vi "LSRS CompleteDrive.vi"() -> ()   [LabVIEW 2017]
uses:
  <vilib>/Rock Robotics/Network Tables/NT Write Numeric Array.vi
panel:
  in  "Error In":errorcluster
  out "Error Out":errorcluster
  out "Right Front Motor Output":dbl
  out "Right Back Motor Output":dbl
  out "Left Front Motor Output":dbl
  out "Left Back Motor Output":dbl
  in  "X":dbl
  in  "Y":dbl
  in  "Z":dbl
  in  "Robot Width":dbl=28.5
  in  "Robot Length":dbl=33.5
  in  "Robot Centric?":bool=TRUE
  in  "Rot. Point X":dbl
  in  "Rot. Point Y":dbl
  in  "Autonomous?":bool
  in  "Yaw":dbl
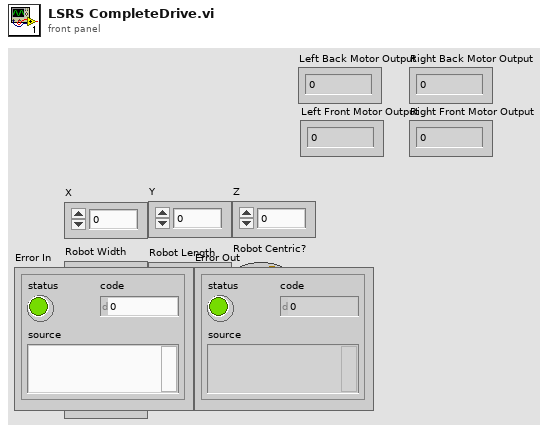
[diagram p1: front panel]
types:
  T1 = typedef "WPI_MotorControlDeviceRef.ctl" = cluster{"DeviceStatus":errorcluster, "Type":T2, "PWM":cluster{"PWM Channel":T3, "DeadBand":T4}, "CAN":cluster{"Device Number":u8, "SetOutput VI Ref":variant, "GetOutput VI Ref":variant, "Enable VI Ref":variant, "Disable VI Ref":variant, "Data":variant}, "Invert":bool, "DIO PWM":cluster{"PWM \"Enable\" Channel":T3, "DIOChannel":T5, "PWM Rate":dbl}}
  T2 = typedef "WPI_MotorControlType.ctl" = enum16{"PWM", "CAN", "DIO PWM"}
  T3 = typedef "FPGA_DIOPWMChannel.ctl" = enum8{"PWM 0", "PWM 1", "PWM 2", "PWM 3", "PWM 4", "PWM 5", "PWM 6", "PWM 7", "PWM 8", "PWM 9", "PWM MXP 0", "PWM MXP 1", "PWM MXP 2", "PWM MXP 3", "PWM MXP 4", "PWM MXP 5", "PWM MXP 6", "PWM MXP 7", "PWM MXP 8", "PWM MXP 9", "Invalid"}
  T4 = typedef "WPI_PWMDeadband.ctl" = cluster{"Name":string, "maxPositivePwm":i32, "minPositivePwm":i32, "centerPwm":i32, "maxNegativePwm":i32, "minNegativePwm":i32, "angularRange":u16}
  T5 = typedef "FPGA_DIOChannel.ctl" = enum8{"DIO 0", "DIO 1", "DIO 2", "DIO 3", "DIO 4", "DIO 5", "DIO 6", "DIO 7", "DIO 8", "DIO 9", "DIO MXP 0", "DIO MXP 1", "DIO MXP 2", "DIO MXP 3", "DIO MXP 4", "DIO MXP 5", "DIO MXP 6", "DIO MXP 7", "DIO MXP 8", "DIO MXP 9", "DIO MXP 10", "DIO MXP 11", "DIO MXP 12", "DIO MXP 13", "DIO MXP 14", "DIO MXP 15", "SPI Port CS1", "SPI Port CS2", "SPI Port CS3", "SPI Port MISO", "SPI Port MOSI", "Invalid"}
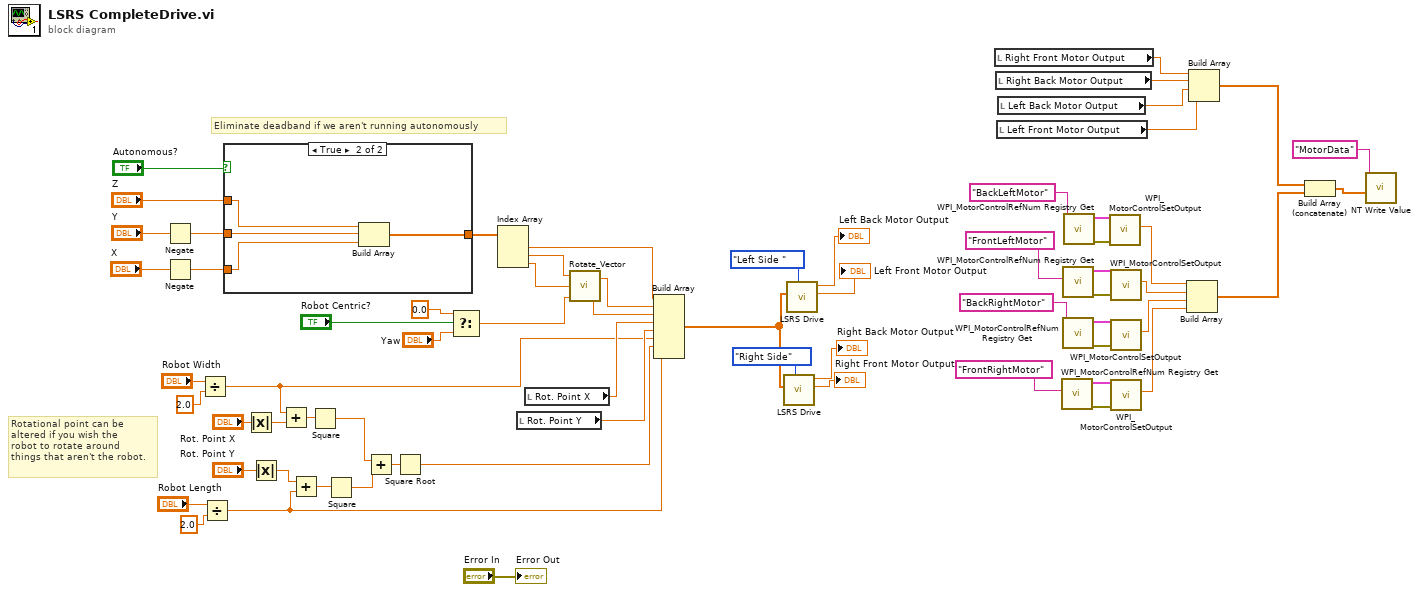
[diagram p0: block diagram]
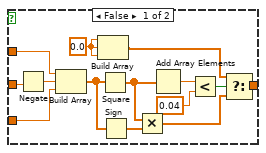
[diagram p2: hidden frame]
diagram:
  # "Rotational point can be \naltered if you wish the \nrobot to rotate around \nthings that aren't the robot."
  # "Eliminate deadband if we aren't running autonomously"
  n1 = Negate(x="Y") -> (-x=w65:dbl)
  n2 = Negate(x="X") -> (-x=w66:dbl)
  n3 = Divide(x="Robot Width", y=2.0) -> (x/y=w35:dbl)
  n4 = Divide(x="Robot Length", y=2.0) -> (x/y=w33:dbl)
  n5 = case shown="True" "Autonomous?" {
    tunnel: w65 -> [w70 w83]
    tunnel: [w69 w81] -> w46
    tunnel: "Z" -> [w68 w84]
    tunnel: w66 -> [w67 w82]
    frame False {
      w76 = 0.0 ("element")
      n6 = Negate(x=w70) -> (-x=w72:dbl)
      n7 = Build Array(w68, w72, w67) -> (w75:dbl[])
      n8 = Build Array(w76, w76, w76) -> (w77:dbl[])
      n9 = Square(x=w75) -> (x^2=w73:dbl[])
      n10 = Sign(1:w75) -> (0:w74:dbl[])
      n11 = Multiply(x=w73, y=w74) -> (x*y=w71:dbl[])
      n12 = Add Array Elements(numeric array=w73) -> (sum=w80:dbl)
      n13 = Less?(x=w80, y=0.04 ("x")) -> (x < y?=w78:bool)
      n14 = Select(t=w77, s=w78, f=w71) -> (s? t:f=w69:dbl[])
    }
    frame True {
      n15 = Build Array(w84, w83, w82) -> (w81:dbl[])
    }
  }
  n16 = Absolute Value(x="Rot. Point X") -> (abs(x)=w56:dbl)
  n17 = Absolute Value(x="Rot. Point Y") -> (abs(x)=w59:dbl)
  n18 = Add(x=w35, y=w56) -> (x+y=w57:dbl)
  n19 = Add(x=w59, y=w33) -> (x+y=w58:dbl)
  n20 = Square(x=w57) -> (x^2=w61:dbl)
  n21 = Square(x=w58) -> (x^2=w60:dbl)
  n22 = Add(x=w61, y=w60) -> (x+y=w62:dbl)
  n23 = Square Root(x=w62) -> (sqrt(x)=w34:dbl)
  n24 = Select(t=0.0, s="Robot Centric?", f="Yaw") -> (s? t:f=w44:dbl)
  n25 = Index Array(array=w46) -> (element #1=w40:dbl, element #2=w42:dbl, element #3=w43:dbl)  [unwired: 3 in]
  n26 = local read "Rot. Point Y"() -> (w36:dbl)
  n27 = local read "Rot. Point X"() -> (w37:dbl)
  n28 = call "Rotate_Vector.vi"("Angle"=w44, "X"=w43, "Y"=w42) -> ("X'"=w38:dbl, "Y'"=w39:dbl)
  n29 = Build Array(w40, w39, w38, w37, w36, w35, w34, w33) -> (w32:dbl[])
  n30 = call "LSRS Drive.vi"("Drive Side"=enum16{"Right Side", "Left Side "}."Right Side", "Inputs"=w32) -> ("Front Motor Output"=→"Right Front Motor Output":dbl, "Back Motor Output"=→"Right Back Motor Output":dbl)  [unwired: 7 in, 1 out]
  n31 = call "LSRS Drive.vi"("Drive Side"=enum16{"Right Side", "Left Side "}."Left Side ", "Inputs"=w32) -> ("Front Motor Output"=→"Left Front Motor Output":dbl, "Back Motor Output"=→"Left Back Motor Output":dbl)  [unwired: 7 in, 1 out]
  n32 = local read "Right Front Motor Output"() -> (w9:dbl)
  n33 = local read "Right Back Motor Output"() -> (w8:dbl)
  n34 = local read "Left Front Motor Output"() -> (w6:dbl)
  n35 = local read "Left Back Motor Output"() -> (w7:dbl)
  n36 = call <vilib>:"WPI_MotorControlRefNum Registry Get.vi"("refnum name"="FrontRightMotor") -> ("error out"=w15:errorcluster, "MotorControlDevRef"=w14:T1)  [unwired: 9 in]
  n37 = call <vilib>:"WPI_MotorControlRefNum Registry Get.vi"("refnum name"="FrontLeftMotor") -> ("error out"=w19:errorcluster, "MotorControlDevRef"=w18:T1)  [unwired: 9 in]
  n38 = call <vilib>:"WPI_MotorControlRefNum Registry Get.vi"("refnum name"="BackRightMotor") -> ("error out"=w17:errorcluster, "MotorControlDevRef"=w16:T1)  [unwired: 9 in]
  n39 = call <vilib>:"WPI_MotorControlRefNum Registry Get.vi"("refnum name"="BackLeftMotor") -> ("error out"=w21:errorcluster, "MotorControlDevRef"=w20:T1)  [unwired: 9 in]
  n40 = call <vilib>:"WPI_MotorControlSetOutput.vi"("error in (no error)"=w21, "MotorControlDevRef"=w20) -> ("Motor Output"=w13:dbl)  [unwired: 7 in, 2 out]
  n41 = call <vilib>:"WPI_MotorControlSetOutput.vi"("error in (no error)"=w19, "MotorControlDevRef"=w18) -> ("Motor Output"=w12:dbl)  [unwired: 7 in, 2 out]
  n42 = call <vilib>:"WPI_MotorControlSetOutput.vi"("error in (no error)"=w17, "MotorControlDevRef"=w16) -> ("Motor Output"=w11:dbl)  [unwired: 7 in, 2 out]
  n43 = call <vilib>:"WPI_MotorControlSetOutput.vi"("error in (no error)"=w15, "MotorControlDevRef"=w14) -> ("Motor Output"=w10:dbl)  [unwired: 7 in, 2 out]
  n44 = Build Array(w13, w12, w11, w10) -> (w4:dbl[])
  n45 = Build Array(w9, w8, w7, w6) -> (w5:dbl[])
  n46 = Build Array (concatenate)(w5, w4) -> (w3:dbl[])
  n47 = call-poly <vilib>:"NT Write Value.vi"("Numeric Array"=w3, "Name"="MotorData") -> ()  [unwired: 9 in, 1 out]
  "Error Out" <- "Error In"
